vi "MT Calculate BER After Trigger (PN Sequence).vi"(0 "input bit stream":i8[](array[numeric]), 5 "PN sequence order (9)":i32=9, 7 "BER trigger threshold (0.1)":dbl=0.1 format="%.4f", 9 "confidence (0.95)":dbl=0.95 format="%.4f", 11 "error in (no error)":errorcluster, 13 "reset? (T)":bool=TRUE) -> (4 "BER":dbl format="%.4f", 6 "accumulated BER":dbl format="%.4f", 8 "trigger found?":bool, 10 "trigger found index (bits)":u32, 15 "error out":errorcluster)   [LabVIEW 2020, in "niDMT.lvlib"]
doc: "This polymorphic instance calculates the average BER against a Galois PN sequence. The sequence must be the same as the PN sequence generated by the Galois instance of the MT Generate Bits (poly) VI with a matching PN order. All subsequent iterations of the VI use a continuation of the same PN sequence until <B>reset?</B> is set to TRUE."
uses:
  <vilib>/addons/Modulation/niDMT.lvlib
  <vilib>/addons/Modulation/niAMT.lvlib
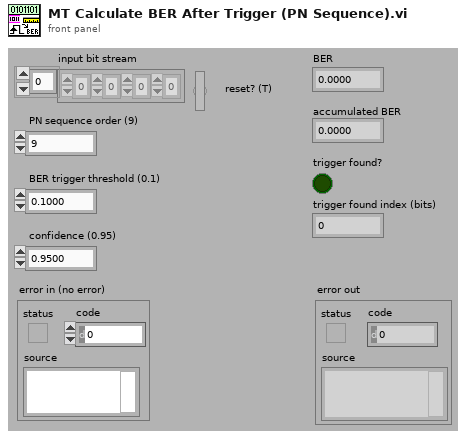
[diagram p1: front panel]
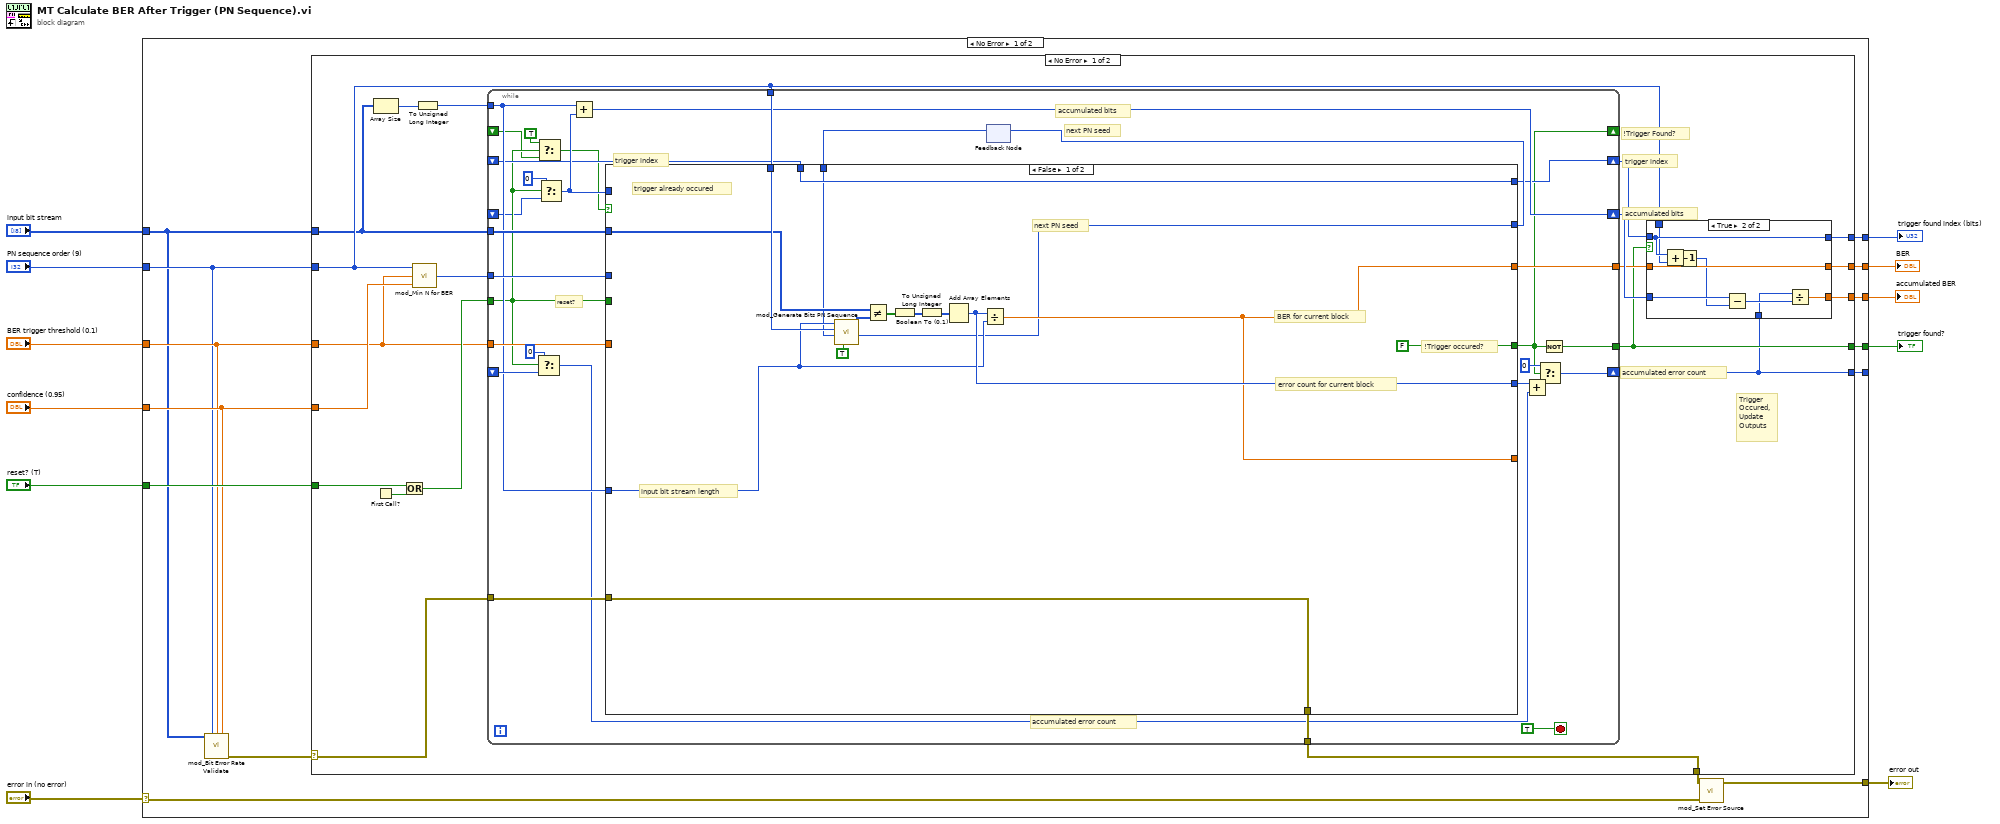
[diagram p0: block diagram]
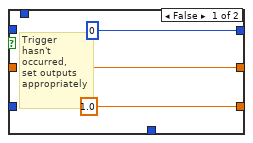
[diagram p2: hidden frame]
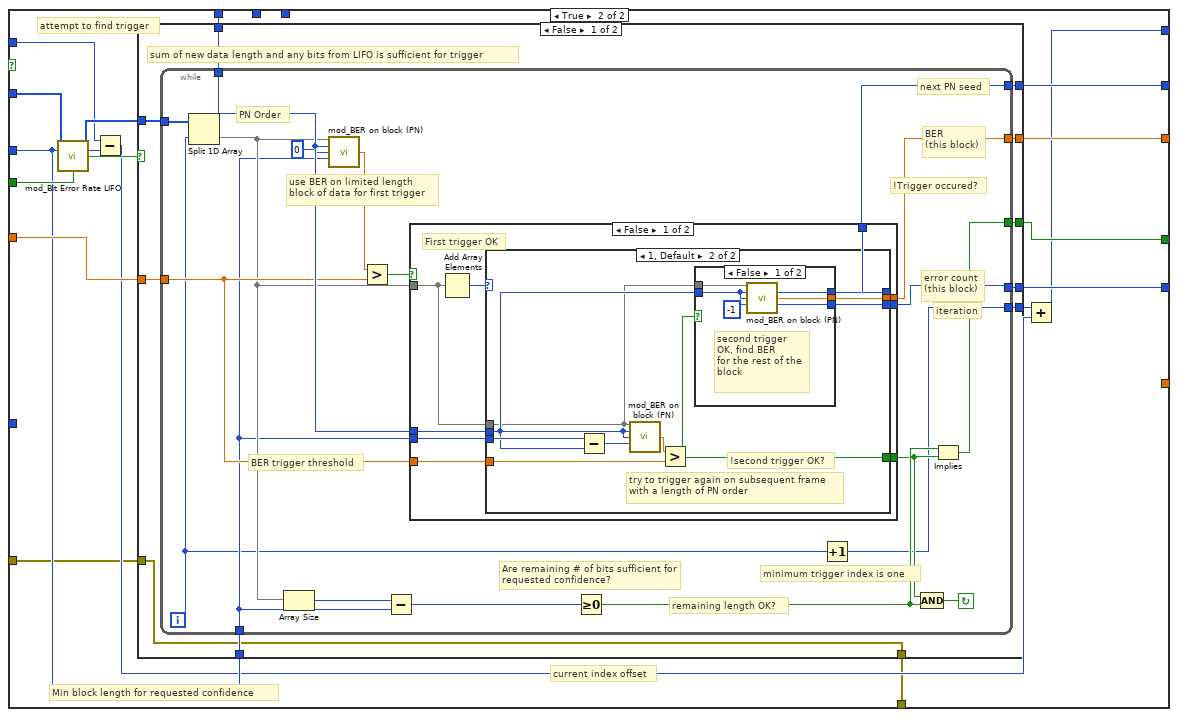
[diagram p3: hidden frame]
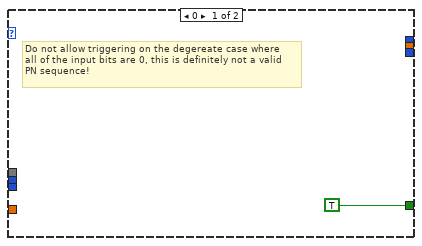
[diagram p4: hidden frame]
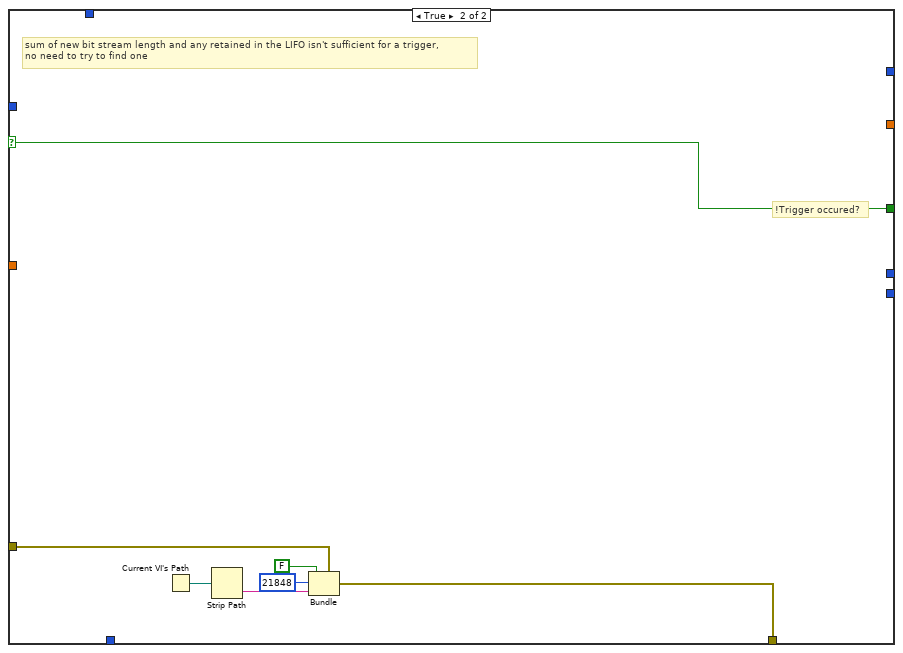
[diagram p7: hidden frame]
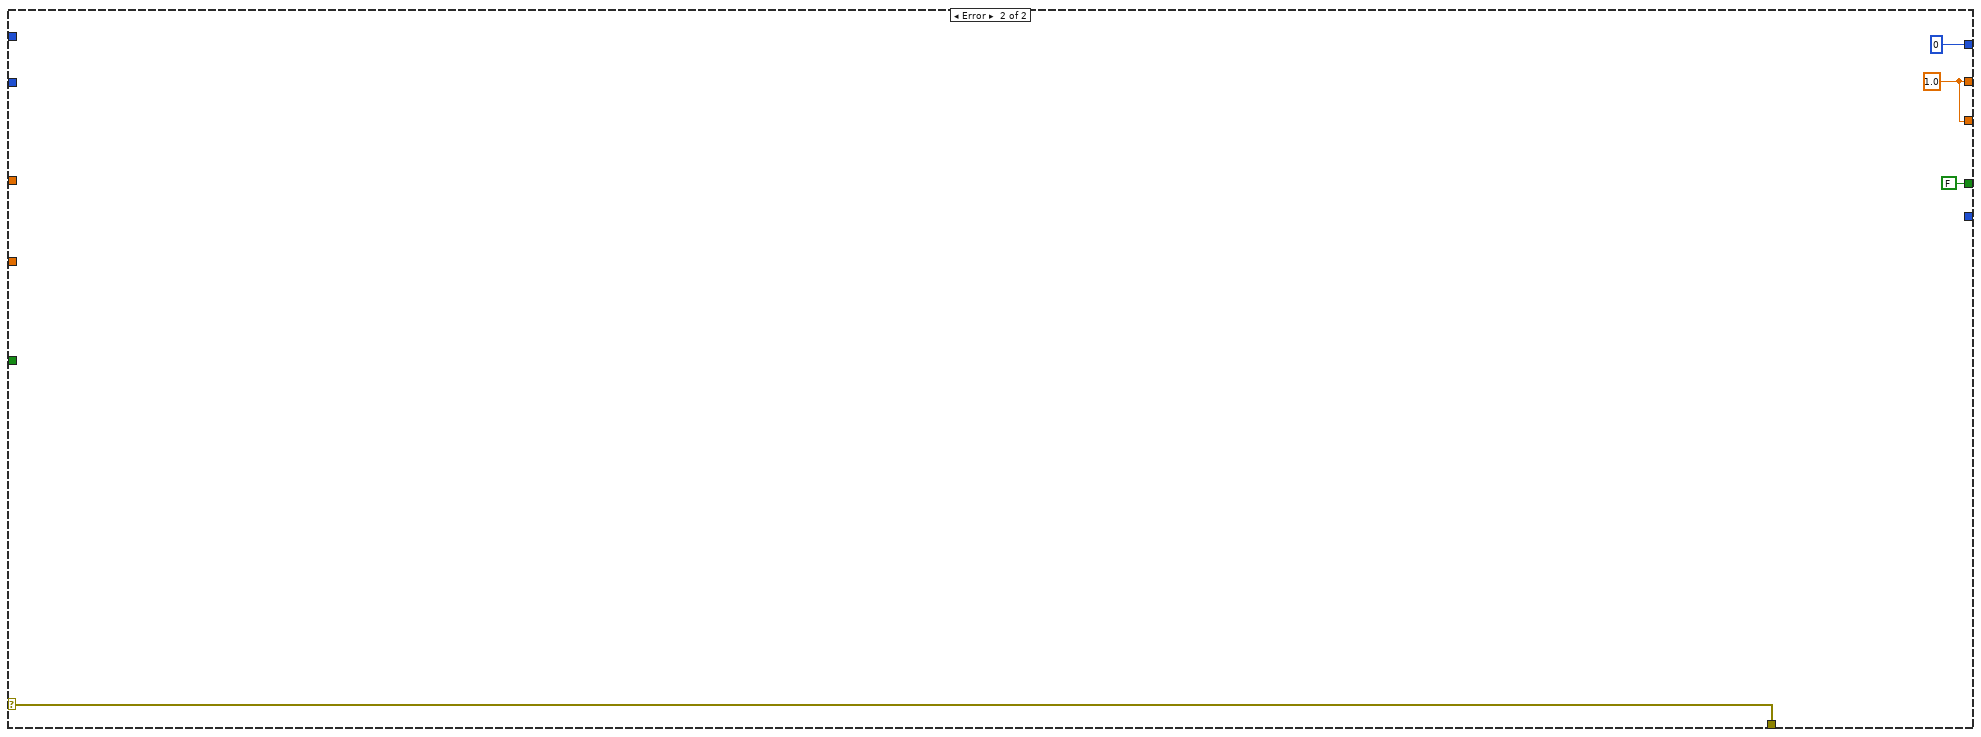
[diagram p8: hidden frame]
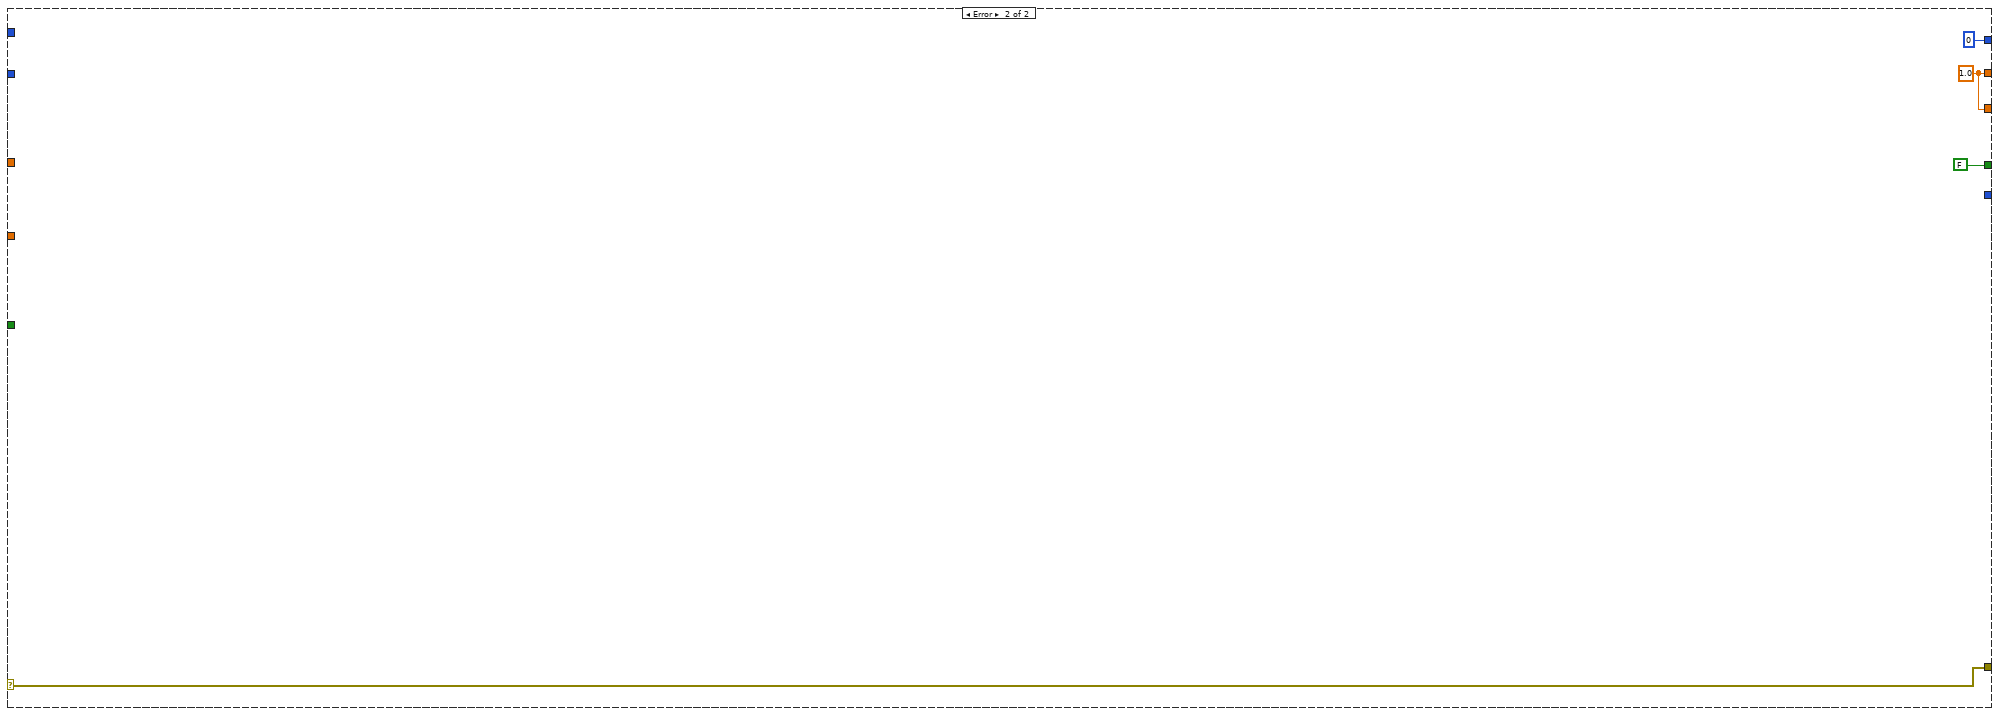
[diagram p9: hidden frame]
diagram:
  n1 = case shown="No Error" "error in (no error)" {
    selector: "error in (no error)" -> [w16 w190]
    tunnel: "reset? (T)" -> [w23 _]
    tunnel: "PN sequence order (9)" -> [w20 _]
    tunnel: "BER trigger threshold (0.1)" -> [w21 _]
    tunnel: "input bit stream" -> [w19 _]
    tunnel: [w25 w189] -> w8
    tunnel: "confidence (0.95)" -> [w22 _]
    tunnel: [w24 w190] -> w6
    tunnel: [w15 w189] -> w3
    tunnel: [w14 u32 0 ("t")] -> w2
    tunnel: [w13 FALSE] -> w1
    tunnel: [w12 _] -> _
    frame No Error {
      n2 = call <vilib>:"mod_Bit Error Rate Validate.vi"("Input Bit Stream"=w19, "PN Sequence Order (9)"=w20, "BER Sync Threshold (0.2)"=w21, "confidence (0.95)"=w22) -> ("error out"=w18:errorcluster)  [unwired: 1 in, 10 out]
      n3 = case shown="No Error" w18 {
        selector: w18 -> [w28 w186]
        tunnel: w20 -> [w32 _]
        tunnel: w21 -> [w33 _]
        tunnel: w19 -> [w30 _]
        tunnel: [w39 w185] -> w25
        tunnel: w22 -> [w34 _]
        tunnel: w23 -> [w42 _]
        tunnel: [w27 w186] -> w17
        tunnel: [w37 w185] -> w15
        tunnel: [w36 u32 0 ("t")] -> w14
        tunnel: [w35 FALSE] -> w13
        tunnel: [w26 _] -> w12
        frame No Error {
          # "Trigger\nOccured,\nUpdate\nOutputs"
          # "!Trigger Found?"
          # "accumulated error count"
          # "trigger index"
          # "accumulated bits"
          n4 = Array Size(array=w30) -> (size(s)=w29:i32)
          n5 = First Call?() -> (First Call?: T/F=w44:bool)
          n6 = Or(x=w42, y=w44) -> (x .or. y?=w43:bool)
          n7 = call <vilib>:"mod_Min N for BER.vi"("confidence"=w34, "threshold"=w33, "PN sequence order"=w32) -> ("min N"=w31:i32)
          n8 = To Unsigned Long Integer(number=w29) -> (unsigned 32bit integer=w38:u32)
          n9 = while {
            shift-right: [w69] -> w41
            shift-left: _ -> [w66]
            tunnel: w43 -> [w65]
            tunnel: w30 -> [w79]
            tunnel: w31 -> [w85]
            tunnel: w32 -> [w84]
            tunnel: w33 -> [w82]
            shift-right: [w71] -> w45
            shift-left: _ -> [w59]
            tunnel: [w81] -> w40
            shift-right: [w77] -> w26
            shift-left: _ -> [w73]
            tunnel: w38 -> [w70]
            tunnel: [w68] -> w35
            shift-right: [w67] -> _
            shift-left: _ -> [w64]
            tunnel: w28 -> [w61]
            tunnel: [w60] -> w27
            stop <- TRUE stop-if-true
            # "accumulated error count"
            # "accumulated bits"
            # "next PN seed"
            # "reset?"
            # "trigger index"
            n10 = Select(t=u32 0, s=w65, f=w73) -> (s? t:f=w58:u32)
            n11 = Select(t=TRUE, s=w65, f=w64) -> (s? t:f=w62:bool)
            n12 = Select(t=u32 0, s=w65, f=w59) -> (s? t:f=w72:u32)
            n13 = Add(x=w70, y=w72) -> (x+y=w71:u32)
            n14 = feedback #1() -> (w75:u32)  [unwired: 1 out]
            n15 = case shown="False" w62 {
              tunnel: w79 -> [w97 w118]
              tunnel: w85 -> [_ w114]
              tunnel: w65 -> [_ w119]
              tunnel: w84 -> [w99 w117]
              tunnel: [w87 w116] -> w83
              tunnel: w82 -> [_ w115]
              tunnel: [w95 w113] -> w81
              tunnel: w72 -> [_ w106]
              tunnel: w66 -> [w98 _]
              tunnel: [w98 w104] -> w69
              tunnel: [FALSE w111] -> w67
              tunnel: [w100 w110] -> w57
              tunnel: w75 -> [w88 _]
              tunnel: w70 -> [w94 _]
              tunnel: w61 -> [w96 w103]
              tunnel: [w96 w102] -> w60
              tunnel: [w95 _] -> _
              frame False {
                # "input bit stream length"
                # "!Trigger occured?"
                # "BER for current block"
                # "error count for current block"
                # "trigger already occured"
                # "next PN seed"
                n16 = call <vilib>:"mod_Generate Bits PN Sequence.vi"("Reset? (T)"=TRUE, "seed in (0xD6BF7DF2)"=w88, "PN Sequence Order (9)"=w99, "Total Bits"=w94) -> ("seed out"=w87:u32, "Output Bit Stream"=w93:i8[])  [unwired: 6 out]
                n17 = Not Equal?(x=w97, y=w93) -> (x != y?=w90:bool[])
                n18 = Boolean To (0,1)(Boolean=w90) -> (0, 1=w91:i16[])
                n19 = To Unsigned Long Integer(number=w91) -> (unsigned 32bit integer=w89:u32[])
                n20 = Add Array Elements(numeric array=w89) -> (sum=w100:u32)
                n21 = Divide(x=w100, y=w94) -> (x/y=w95:dbl)
              }
              frame True {
                # "Min block length for requested confidence"
                # "current index offset"
                # "attempt to find trigger"
                n22 = call <vilib>:"mod_Bit Error Rate LIFO.vi"("input bit stream"=w118, "max buffer length"=w114, "reset"=w119) -> ("output bit stream"=w112:i8[], "Old Buffer Length (Prior to New Bits)"=w107:i32, "Updated Buffer Length less \nthan max length"=w109:bool)  [unwired: 10 out]
                n23 = Subtract(x=w106, y=w107) -> (x-y=w105:u32)
                n24 = case shown="False" w109 {
                  selector: w109 -> [_ w182]
                  tunnel: w117 -> [w129 _]
                  tunnel: [w128 _] -> w116
                  tunnel: w115 -> [w127 _]
                  tunnel: w114 -> [w126 _]
                  tunnel: [w125 _] -> w113
                  tunnel: w112 -> [w124 _]
                  tunnel: [w123 w182] -> w111
                  tunnel: [w122 _] -> w110
                  tunnel: [w121 _] -> w108
                  tunnel: w103 -> [w120 w180]
                  tunnel: [w120 w176] -> w102
                  frame False {
                    # "sum of new data length and any bits from LIFO is sufficient for trigger"
                    n25 = while {
                      tunnel: w129 -> [w143]
                      tunnel: w124 -> [w148]
                      tunnel: [w130] -> w128
                      tunnel: w127 -> [w141]
                      tunnel: w126 -> [w135]
                      tunnel: [w146] -> w125
                      tunnel: [w136] -> w123
                      tunnel: [w132] -> w121
                      tunnel: [w145] -> w122
                      i -> [w133]
                      stop <- w144 continue-if-true
                      # "minimum trigger index is one"
                      # "remaining length OK?"
                      # "BER\n(this block)"
                      # "error count\n(this block)"
                      # "iteration"
                      # "Are remaining # of bits sufficient for requested confidence?"
                      # "BER trigger threshold"
                      # "!Trigger occured?"
                      # "PN Order"
                      # "use BER on limited length\nblock of data for first trigger"
                      # "next PN seed"
                      n26 = Split 1D Array(array=w148, index=w133) -> (second subarray=w139:i8[])  [unwired: 1 out]
                      n27 = Array Size(array=w139) -> (size(s)=w140:i32)
                      n28 = call <vilib>:"mod_BER on block (PN).vi"("bit stream in"=w139, "expected PN sequence order"=w143, "starting index"=0, "length (0 or negative = entire block)"=w135) -> ("BER"=w131:dbl)  [unwired: 11 out]
                      n29 = Greater?(x=w131, y=w141) -> (0:w142:bool)
                      n30 = Subtract(x=w140, y=w135) -> (x-y=w147:i32)
                      n31 = case shown="False" w142 {
                        selector: w142 -> [_ w175]
                        tunnel: w139 -> [w150 _]
                        tunnel: [w156 _] -> w146
                        tunnel: w143 -> [w151 _]
                        tunnel: [w155 _] -> w145
                        tunnel: [w157 _] -> w130
                        tunnel: [w153 w175] -> w137
                        tunnel: w141 -> [w154 _]
                        tunnel: w135 -> [w152 _]
                        frame False {
                          # "First trigger OK"
                          n32 = Add Array Elements(numeric array=w150) -> (sum=w149:i8)
                          n33 = case shown="1, Default" w149 {
                            tunnel: [_ w168] -> w157
                            tunnel: [_ w167] -> w156
                            tunnel: [_ w166] -> w155
                            tunnel: w154 -> [_ w164]
                            tunnel: [TRUE w162] -> w153
                            tunnel: w152 -> [_ w161]
                            tunnel: w151 -> [_ w160]
                            tunnel: w150 -> [_ w159]
                            frame 0 {
                              # "Do not allow triggering on the degereate case where\nall of the input bits are 0, this is definitely not a valid\nPN sequence!"
                            }
                            frame 1, Default {
                              # "!second trigger OK?"
                              # "try to trigger again on subsequent frame\nwith a length of PN order"
                              n34 = Subtract(x=w161, y=w160) -> (x-y=w163:i32)
                              n35 = call <vilib>:"mod_BER on block (PN).vi"("bit stream in"=w159, "expected PN sequence order"=w160, "starting index"=w160, "length (0 or negative = entire block)"=w163) -> ("BER"=w165:dbl)  [unwired: 11 out]
                              n36 = Greater?(x=w165, y=w164) -> (0:w162:bool)
                              n37 = case shown="False" w162 {
                                tunnel: [w174 _] -> w168
                                tunnel: [w173 _] -> w167
                                tunnel: [w172 _] -> w166
                                tunnel: w159 -> [w171 _]
                                tunnel: w160 -> [w169 _]
                                frame False {
                                # "second trigger\nOK, find BER\nfor the rest of the\nblock"
                                n38 = call <vilib>:"mod_BER on block (PN).vi"("bit stream in"=w171, "expected PN sequence order"=w169, "starting index"=w169, "length (0 or negative = entire block)"=-1 ("length")) -> ("next seed"=w174:u32, "BER"=w173:dbl, "number of errors"=w172:u32)  [unwired: 9 out]
                                }
                                frame True {
                                }
                              }
                            }
                          }
                        }
                        frame True {
                        }
                      }
                      n39 = Greater Or Equal To 0?(x=w147) -> (x >= 0?=w138:bool)
                      n40 = Increment(x=w133) -> (x+1=w132:i32)
                      n41 = Compound Arithmetic op=AND(w137, w138) -> (w144:bool)
                      n42 = Implies(1:w137, 2:w138) -> (0:w136:bool)
                    }
                  }
                  frame True {
                    # "!Trigger occured?"
                    # "sum of new bit stream length and any retained in the LIFO isn't sufficient for a trigger,\nno need to try to find one"
                    n43 = Current VI's Path() -> (path=w181:path)
                    n44 = Strip Path(path=w181) -> (name=w178:string)  [unwired: 1 out]
                    n45 = Bundle(cluster=w180, "status"=FALSE, "code"=21848, "source"=w178) -> (w176:errorcluster)
                  }
                }
                n46 = Add(x=w108, y=w105) -> (x+y=w104:u32)
              }
            }
            n47 = feedback-in #1(w83) -> ()
            n48 = Add(x=w57, y=w58) -> (x+y=w78:u32)
            n49 = Select(t=u32 0, s=w67, f=w78) -> (s? t:f=w77:u32)
            n50 = Not(x=w67) -> (.not. x?=w68:bool)
          }
          n51 = case shown="True" w35 {
            tunnel: w45 -> [_ w53]
            tunnel: w26 -> [_ w52]
            tunnel: [w47 w56] -> w37
            tunnel: w41 -> [_ w51]
            tunnel: w40 -> [_ w55]
            tunnel: [w47 w55] -> w39
            tunnel: [u32 0 ("t") w51] -> w36
            tunnel: w32 -> [_ w50]
            frame False {
              w47 = 1.0 ("f")
              # "Trigger\nhasn't \noccurred,\nset outputs\nappropriately"
            }
            frame True {
              n52 = Add(x=w51, y=w50) -> (x+y=w49:u32)
              n53 = Decrement(x=w49) -> (x-1=w48:u32)
              n54 = Subtract(x=w53, y=w48) -> (x-y=w54:u32)
              n55 = Divide(x=w52, y=w54) -> (x/y=w56:dbl)
            }
          }
        }
        frame Error {
          w185 = 1.0
        }
      }
      n56 = call <vilib>:"mod_Set Error Source.vi"("initial error in (no error)"=w16, "final error in (no error)"=w17) -> ("error out"=w24:errorcluster)  [unwired: 3 out]
    }
    frame Error {
      w189 = 1.0
    }
  }
  "BER" <- w8
  "error out" <- w6
  "accumulated BER" <- w3
  "trigger found index (bits)" <- w2
  "trigger found?" <- w1
